vi "RT Main2.vi"() -> ()   [LabVIEW 2019]
uses:
  <vilib>/FPGAPlugInAG/ELVIS III/niLvFpga_Open_ELVIS III.vi
  <vilib>/rvi/interface/common/dynamic/niFpgaDynamicAddResources.vi
  <vilib>/Utility/error.llb/Error Cluster From Error Code.vi
  <vilib>/rvi/errors/niLvFpgaAdjustHostInterfaceError.vi
  <vilib>/rvi/interface/common/niFpgaWaitOnOcc.vi
  <vilib>/FPGAPlugInAG/Dynamic/niLvFpga_Run_Dynamic.vi
  <vilib>/measure/maspectr.llb/FFT Spectrum (Real-Im) for 1 Chan.vi
  <vilib>/FPGAPlugInAG/Dynamic/niLvFpga_Close_Dynamic.vi
  <vilib>/rvi/interface/nirviOpenFPGA/nirviOpenFPGA.xnode
  FPGA-Main2.vi
  <vilib>/rvi/interface/nirviReadWriteControl/nirviReadWriteControl.xnode
  <vilib>/rvi/interface/nirviMethod/nirviMethod.xnode
  <vilib>/rvi/interface/nirviCloseFPGA/nirviCloseFPGA.xnode
  NiFpgaLv.dll
  <vilib>/rvi/interface/Simulation/niFpgaSimulationCallBeginRW.vi
  <vilib>/FPGAPlugInAG/Dynamic/niLvFpga_ConfigureFifo_Dynamic.vi
  <vilib>/rvi/errors/niLvFpgaMergeErrorWithErrorCode.vi
  <vilib>/FPGAPlugInAG/Dynamic/niLvFpga_ReadFifo_Dynamic.vi
  <vilib>/measure/NI_MAPro.lvlib
panel:
  out "波形图表 5":waveform(dbl)(graph)
  out "error out":errorcluster caption="错误输出"
  out "波形图表 4":waveform(dbl)(graph)
  out "波形图表 3":waveform(dbl)(graph)
  in  "停止":bool
  out "波形图表":waveform(dbl)(graph)
  in  "Count(uSec)":u32=10
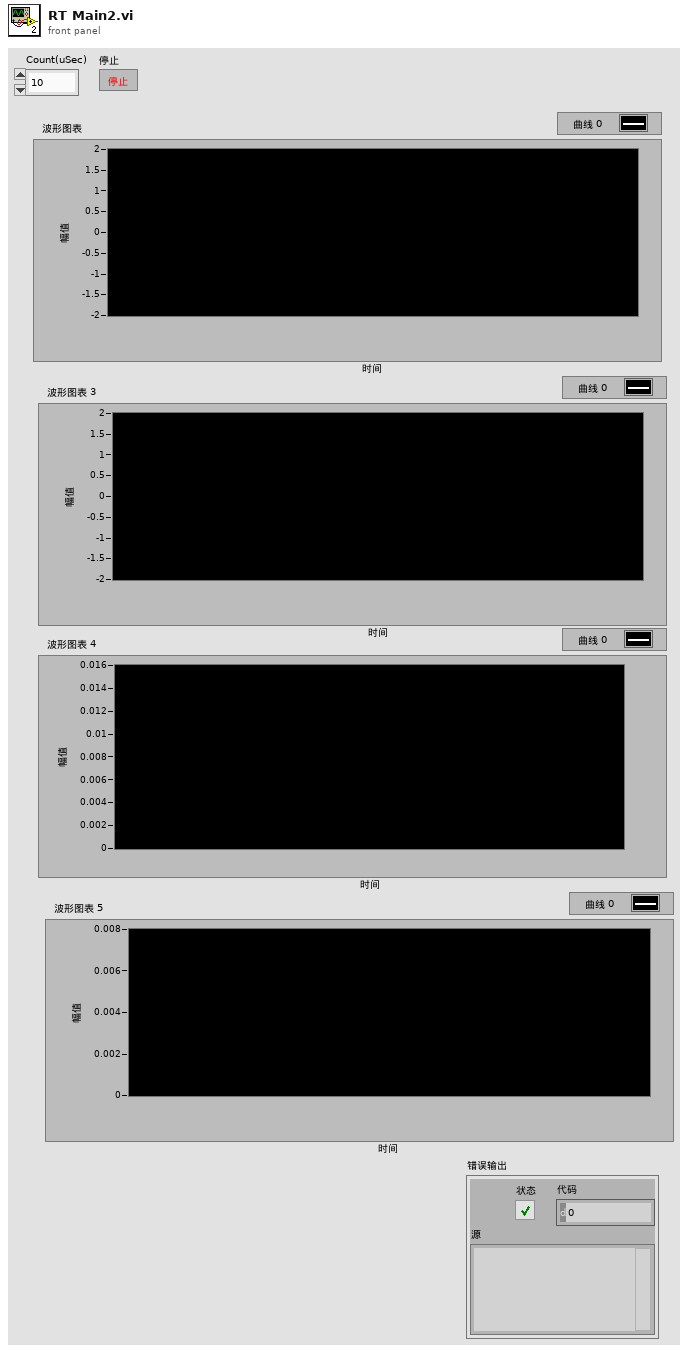
[diagram p1: front panel]
types:
  T1 = cluster{"f0":dbl, "df":dbl, "imaginary part":dbl[]}
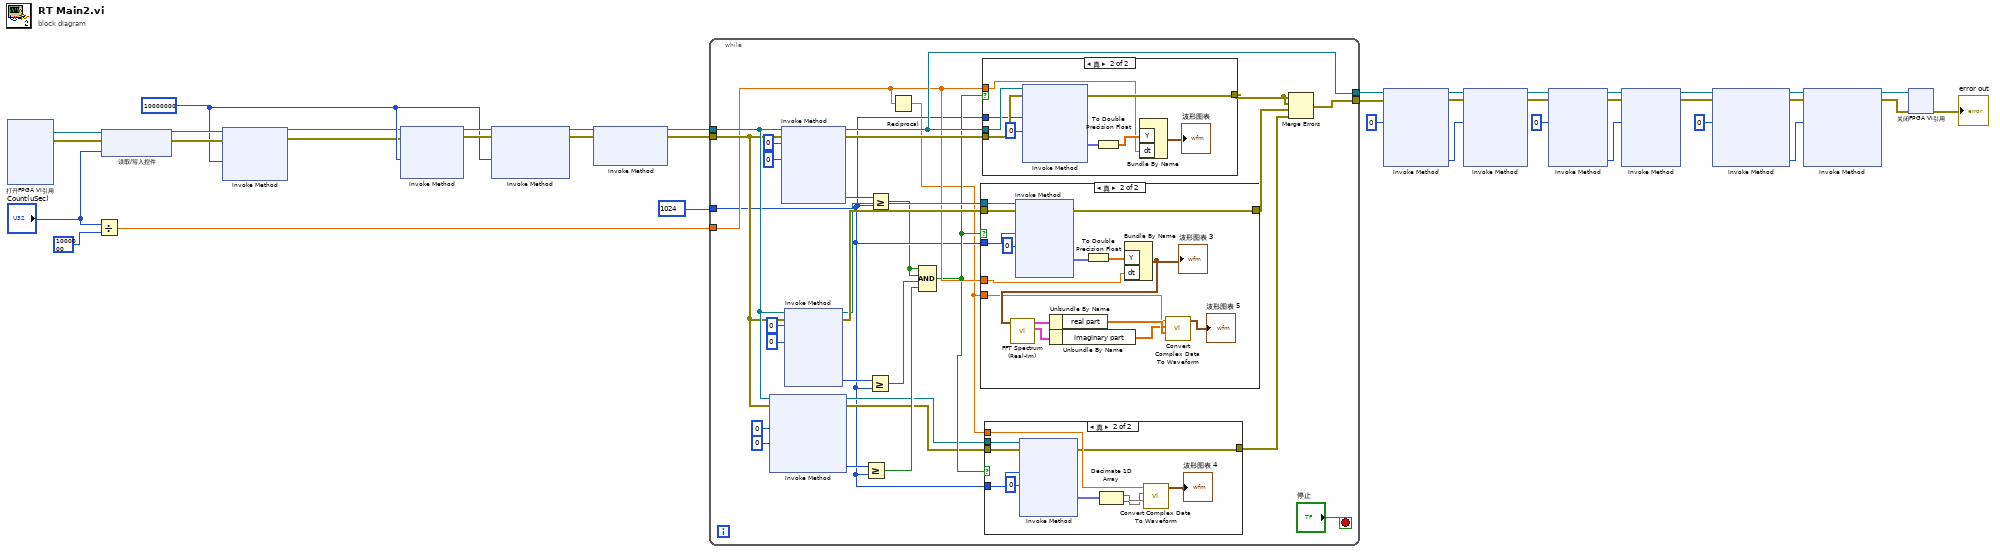
[diagram p0: block diagram]
diagram:
  w30 = u32 10000000 ("请求的深度")
  n1 = xnode "打开FPGA VI引用"() -> ("FPGA VI引用输出"=w37:refnum<k20>, "错误输出"=w38:errorcluster)  [unwired: 2 in]
  n2 = Divide(x="Count(uSec)", y=u32 1000000 ("请求的深度")) -> (x/y=w25:dbl)
  n3 = xnode "读取/写入控件"("FPGA VI引用输入"=w37, "错误输入"=w38, "Count(uSec)"="Count(uSec)") -> ("FPGA VI引用输出"=w35:refnum<k20>, "错误输出"=w36:errorcluster)
  n4 = xnode "Invoke Method"("FPGA VI引用输入"=w35, "错误输入"=w36, "请求的深度"=w30) -> ("FPGA VI引用输出"=w3:refnum<k20>, "错误输出"=w4:errorcluster)  [unwired: 1 out]
  n5 = xnode "Invoke Method"("FPGA VI引用输入"=w3, "错误输入"=w4, "请求的深度"=w30) -> ("FPGA VI引用输出"=w33:refnum<k20>, "错误输出"=w34:errorcluster)  [unwired: 1 out]
  n6 = xnode "Invoke Method"("FPGA VI引用输入"=w33, "错误输入"=w34, "请求的深度"=w30) -> ("FPGA VI引用输出"=w31:refnum<k20>, "错误输出"=w32:errorcluster)  [unwired: 1 out]
  n7 = xnode "Invoke Method"("FPGA VI引用输入"=w31, "错误输入"=w32) -> ("FPGA VI引用输出"=w26:refnum<k20>, "错误输出"=w27:errorcluster)  [unwired: 1 in]
  n8 = while {
    tunnel: w27 -> [w66]
    tunnel: w26 -> [w67]
    tunnel: w25 -> [w54]
    tunnel: u32 1024 -> [w49]
    tunnel: [w58] -> w23
    tunnel: [w57] -> w22
    stop <- "停止" stop-if-true
    n9 = xnode "Invoke Method"("FPGA VI引用输入"=w67, "错误输入"=w66, "元素数量"=u32 0, "超时(ms)"=0) -> ("FPGA VI引用输出"=w50:refnum<k20>, "错误输出"=w51:errorcluster, "剩余元素"=w65:u32)  [unwired: 1 out]
    n10 = xnode "Invoke Method"("FPGA VI引用输入"=w67, "错误输入"=w66, "元素数量"=u32 0, "超时(ms)"=0) -> ("FPGA VI引用输出"=w57:refnum<k20>, "错误输出"=w60:errorcluster, "剩余元素"=w63:u32)  [unwired: 1 out]
    n11 = xnode "Invoke Method"("FPGA VI引用输入"=w67, "错误输入"=w66, "元素数量"=u32 0, "超时(ms)"=0) -> ("FPGA VI引用输出"=w55:refnum<k20>, "错误输出"=w56:errorcluster, "剩余元素"=w64:u32)  [unwired: 1 out]
    n12 = Greater Or Equal?(x=w65, y=w49) -> (x >= y?=w61:bool)
    n13 = Greater Or Equal?(x=w64, y=w49) -> (x >= y?=w62:bool)
    n14 = Greater Or Equal?(x=w63, y=w49) -> (x >= y?=w40:bool)
    n15 = Reciprocal(x=w54) -> (1/x=w39:dbl)
    n16 = Compound Arithmetic op=AND ("复合运算")(w40, w40, w62, w61) -> (w52:bool)
    n17 = case shown="真" w52 {
      tunnel: w56 -> [w79 w94]
      tunnel: w55 -> [_ w93]
      tunnel: w49 -> [_ w92]
      tunnel: w54 -> [_ w88]
      tunnel: [w79 w87] -> w53
      tunnel: w39 -> [_ w81]
      frame False {
      }
      frame True {
        n18 = xnode "Invoke Method"("FPGA VI引用输入"=w93, "错误输入"=w94, "元素数量"=w92, "超时(ms)"=0) -> ("错误输出"=w87:errorcluster, "数据"=w90:fxp<+/-,24,5>[])  [unwired: 2 out]
        n19 = To Double Precision Float(number=w90) -> (double precision float=w89:dbl[])
        n20 = Bundle By Name("Y"=w89, "dt"=w88) -> (w86:waveform(dbl))  [unwired: 1 in]
        "波形图表 3" <- w86
        n21 = call-poly <vilib>:"FFT Spectrum (Real-Im).vi"("time signal"=w86) -> ("imaginary part"=w84:T1, "real part"=w85:cluster{"f0":dbl, "df":dbl, "real part":dbl[]})  [unwired: 6 in, 3 out]
        n22 = Unbundle By Name(w85) -> ("real part"=w83:dbl[])
        n23 = Unbundle By Name(w84) -> ("imaginary part"=w82:dbl[])
        n24 = call "Convert Complex Data To Waveform.vi"("Real Data"=w83, "Imaginary Data"=w82, "Sample Rate (S/s)"=w81) -> ("Waveform"=→"波形图表 5":waveform(dbl))  [unwired: 7 in, 1 out]
      }
    }
    n25 = case shown="真" w52 {
      tunnel: w60 -> [w95 w104]
      tunnel: w57 -> [_ w103]
      tunnel: [w95 w102] -> w41
      tunnel: w54 -> [_ w99]
      tunnel: w49 -> [_ w97]
      frame False {
      }
      frame True {
        n26 = xnode "Invoke Method"("FPGA VI引用输入"=w103, "错误输入"=w104, "元素数量"=w97, "超时(ms)"=0) -> ("错误输出"=w102:errorcluster, "数据"=w101:fxp<+/-,24,5>[])  [unwired: 2 out]
        n27 = To Double Precision Float(number=w101) -> (double precision float=w100:dbl[])
        n28 = Bundle By Name("Y"=w100, "dt"=w99) -> (→"波形图表":waveform(dbl))  [unwired: 1 in]
      }
    }
    n29 = case shown="真" w52 {
      tunnel: w51 -> [w68 w78]
      tunnel: w50 -> [_ w77]
      tunnel: w49 -> [_ w76]
      tunnel: w39 -> [_ w73]
      tunnel: [w68 w71] -> w48
      frame False {
      }
      frame True {
        n30 = xnode "Invoke Method"("FPGA VI引用输入"=w77, "错误输入"=w78, "元素数量"=w76, "超时(ms)"=0) -> ("错误输出"=w71:errorcluster, "数据"=w74:fxp<+/-,24,5>[])  [unwired: 2 out]
        n31 = Decimate 1D Array(w74) -> (w70:fxp<+/-,24,5>[], w69:fxp<+/-,24,5>[])
        n32 = call "Convert Complex Data To Waveform.vi"("Real Data"=w70, "Imaginary Data"=w69, "Sample Rate (S/s)"=w73) -> ("Waveform"=→"波形图表 4":waveform(dbl))  [unwired: 7 in, 1 out]
      }
    }
    n33 = Merge Errors(w41, w41, w53, w48) -> (w58:errorcluster)
  }
  n34 = xnode "Invoke Method"("FPGA VI引用输入"=w22, "错误输入"=w23, "元素数量"=u32 0) -> ("FPGA VI引用输出"=w20:refnum<k20>, "错误输出"=w21:errorcluster, "剩余元素"=w10:u32)  [unwired: 1 in, 1 out]
  n35 = xnode "Invoke Method"("FPGA VI引用输入"=w20, "错误输入"=w21, "元素数量"=w10) -> ("FPGA VI引用输出"=w1:refnum<k20>, "错误输出"=w2:errorcluster)  [unwired: 1 in, 2 out]
  n36 = xnode "Invoke Method"("FPGA VI引用输入"=w1, "错误输入"=w2, "元素数量"=u32 0) -> ("FPGA VI引用输出"=w16:refnum<k20>, "错误输出"=w19:errorcluster, "剩余元素"=w8:u32)  [unwired: 1 in, 1 out]
  n37 = xnode "Invoke Method"("FPGA VI引用输入"=w16, "错误输入"=w19, "元素数量"=w8) -> ("FPGA VI引用输出"=w15:refnum<k20>, "错误输出"=w18:errorcluster)  [unwired: 1 in, 2 out]
  n38 = xnode "Invoke Method"("FPGA VI引用输入"=w15, "错误输入"=w18, "元素数量"=u32 0) -> ("FPGA VI引用输出"=w14:refnum<k20>, "错误输出"=w17:errorcluster, "剩余元素"=w9:u32)  [unwired: 1 in, 1 out]
  n39 = xnode "Invoke Method"("FPGA VI引用输入"=w14, "错误输入"=w17, "元素数量"=w9) -> ("FPGA VI引用输出"=w12:refnum<k20>, "错误输出"=w13:errorcluster)  [unwired: 1 in, 2 out]
  n40 = xnode "关闭FPGA VI引用"("FPGA VI引用输入"=w12, "错误输入"=w13) -> ("错误输出"=→"error out":errorcluster)
